vi "Configure Measurement (Spectrum Emission Mask - Reference).vi"(0 "VISA resource name":refnum<visa-resource-name>, 1 "Auto Total Power Reference (T: Enable)":bool=TRUE, 5 "Measurement Type (0: Total Power Reference)":i32(ring) items=["Total Power Reference", "PSD Reference"], 9 "Integration Bandwidth (3.48E+6 Hz)":dbl=3480000.0, 11 "error in (no error)":errorcluster, 12 "Total Power Reference (-72 dBm)":dbl=-72.0) -> (4 "VISA resource name out":refnum<visa-resource-name>, 15 "error out":errorcluster)   [LabVIEW 2022 SP3, in "Agilent N934X Series.lvlib"]
doc: "Configure the Integration Bandwidth and Reference settings in either Total Pwr or PSD measurement mode under Spectrum Emission Mask measurement.\n\nNote:\nThis VI is only applicable for N9321C, N9322C, N9323C, N9324C models"
uses:
  <instrlib>/Agilent N934X Series/Agilent N934X Series.lvlib
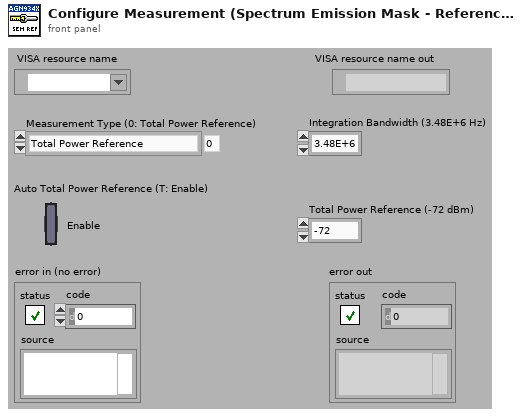
[diagram p1: front panel]
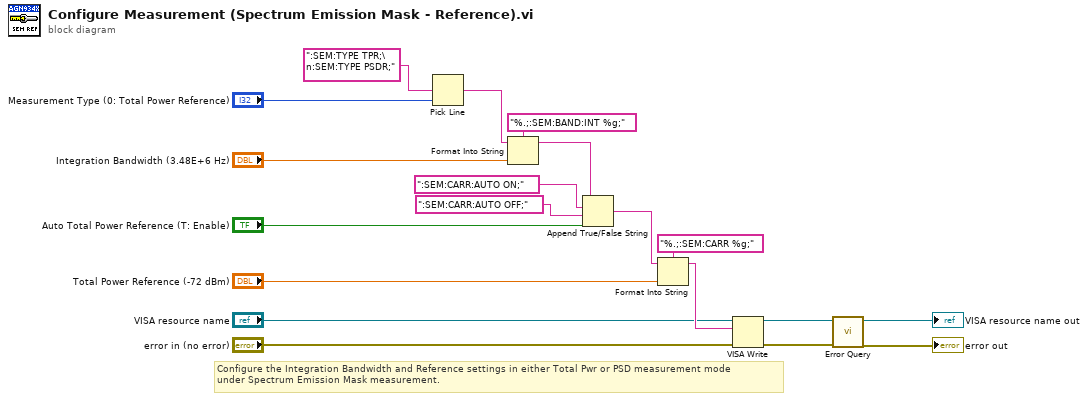
[diagram p0: block diagram]
diagram:
  # "Configure the Integration Bandwidth and Reference settings in either Total Pwr or PSD measurement mode \nunder Spectrum Emission Mask measurement."
  n1 = Pick Line(multi-line string=":SEM:TYPE TPR;\n:SEM:TYPE PSDR;", line index="Measurement Type (0: Total Power Reference)") -> (output string=w17:string)  [unwired: 1 in]
  n2 = Format Into String(format string="%.;:SEM:BAND:INT %g;", initial string=w17, "Integration Bandwidth (3.48E+6 Hz)") -> (resulting string=w14:string)  [unwired: 1 in, 1 out]
  n3 = Append True/False String(1:"Auto Total Power Reference (T: Enable)", 2:":SEM:CARR:AUTO OFF;", 3:":SEM:CARR:AUTO ON;", 4:w14) -> (0:w10:string)
  n4 = Format Into String(format string="%.;:SEM:CARR %g;", initial string=w10, "Total Power Reference (-72 dBm)") -> (resulting string=w7:string)  [unwired: 1 in, 1 out]
  n5 = VISA Write(VISA resource name="VISA resource name", write buffer=w7, error in (no error)="error in (no error)") -> (VISA resource name out=w4:refnum<visa-resource-name>, error out=w3:errorcluster)  [unwired: 1 out]
  n6 = call <instrlib>:"Error Query.vi"("error in (no error)"=w3, "VISA resource name"=w4) -> ("error out"=→"error out":errorcluster, "VISA resource name out"=→"VISA resource name out":refnum<visa-resource-name>)  [unwired: 6 in, 2 out]
